vi "FDG Def_Start_Results.vi"(0 "System no.":i32=1 min=1 step=1, 1 "Board":i32=1 min=1 max=5 step=1, 2 "Routinename":string, 5 "error in":errorcluster, 6 "Treshold level":dbl=1.0 format="%.3f", 7 "Frequency settings":cluster{"Set frequency?":bool, "Frequency":dbl}={"Set frequency?"=FALSE, "Frequency"=10.0} {"Frequency" format="%.3f"}, 8 "Velocity settings":cluster{"Set velocity?":bool, "Velocity":dbl}={"Set velocity?"=FALSE, "Velocity"=0.1} {"Velocity" format="%.4f"}, 9 "Max. direction changes settings":T3={"Set max. dir. changes?"=FALSE, "Max. dir. changes"=10}, 10 "Speed factor settings":T4={"Set speed factor?"=FALSE, "Speed factor"=0.25} {"Speed factor" format="%.4f"}, 11 "Speed offset settings":T2={"Set speed offset?"=FALSE, "Speed offset"=0.05} {"Speed offset" format="%.4f"}, 12 "Stop refnum":refnum<vi>, 13 "Polling time in ms":u32=1) -> (14 "Scan successful?":bool, 15 "Level at max. pos.":dbl=1.0 format="%.4f", 16 "Pos. at max. information":string, 19 "error out":errorcluster)   [LabVIEW 2026]
doc: "Defines a fast alignment gradient search routine, starts search, waits until search has finished and queries results. If Stop refnum or Local stop is TRUE, VI sends #24 and stops."
panel:
  in  "Amplitude settings":T1={"Min amplitude"=0.4, "Set min. amplitude?"=FALSE, "Max amplitude"=0.8, "Set max. amplitude?"=FALSE} {"Max amplitude" format="%.4f"; "Min amplitude" format="%.4f"}
  in  "Axis settings":cluster{"Scan axis":string, "Step axis":string}
  in  "Local stop":bool
  # "Defines fast gradient scan, starts scan, waits until scan has finished and queries results.  If Stop refnum or Local stop is TRUE, VI sends #24 and stops."
  # "If Yes:"
  # "If Yes:"
  # "If Yes:"
  # "If Yes:"
  # "If Yes:"
  # "If Yes:"
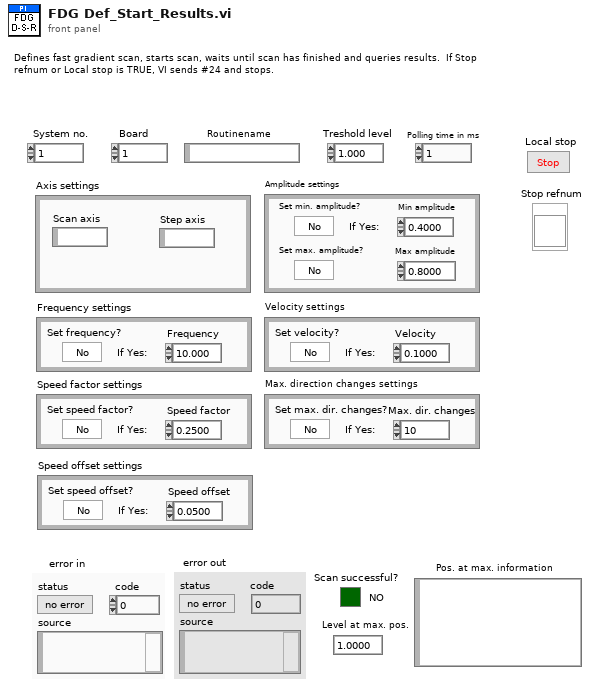
[diagram p1: front panel]
types:
  T1 = cluster{"Min amplitude":dbl, "Set min. amplitude?":bool, "Max amplitude":dbl, "Set max. amplitude?":bool}
  T2 = cluster{"Set speed offset?":bool, "Speed offset":dbl}
  T3 = cluster{"Set max. dir. changes?":bool, "Max. dir. changes":i32}
  T4 = cluster{"Set speed factor?":bool, "Speed factor":dbl}
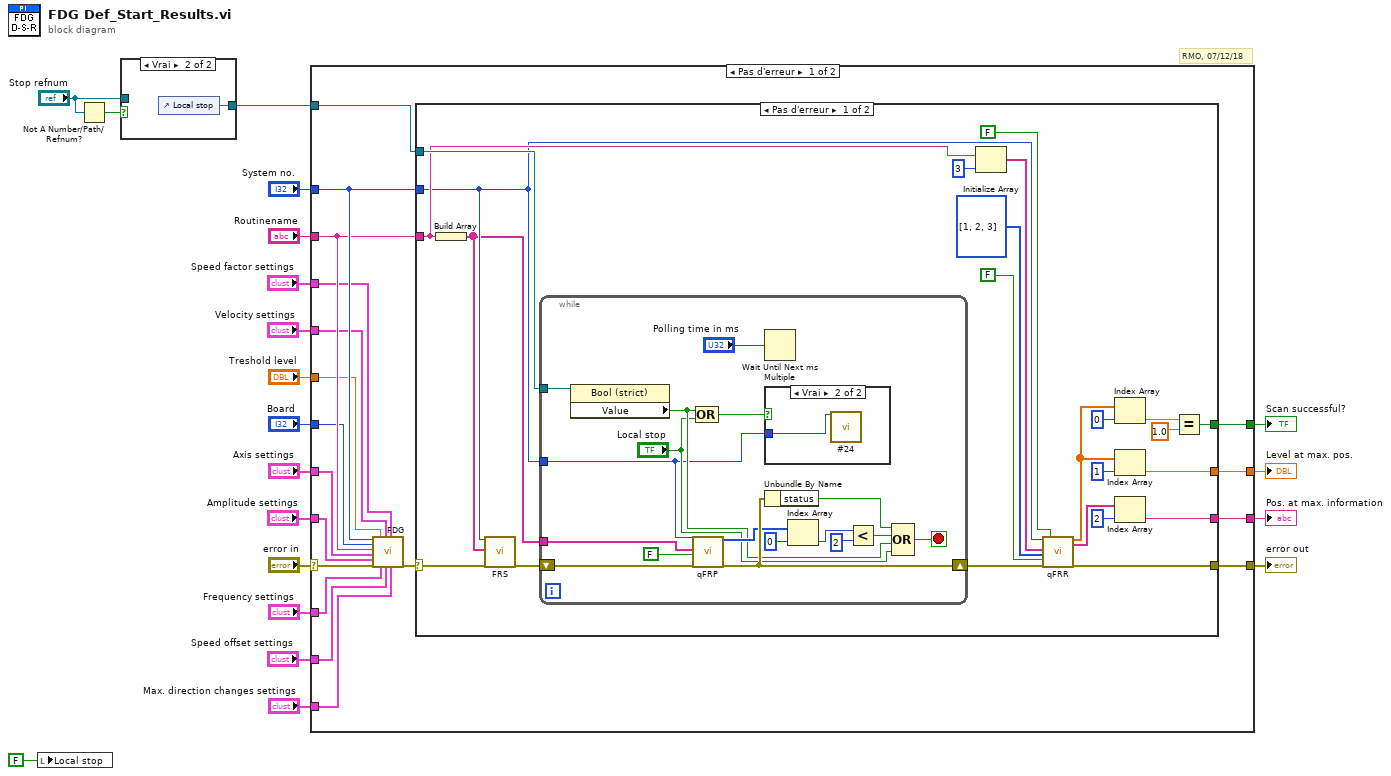
[diagram p0: block diagram]
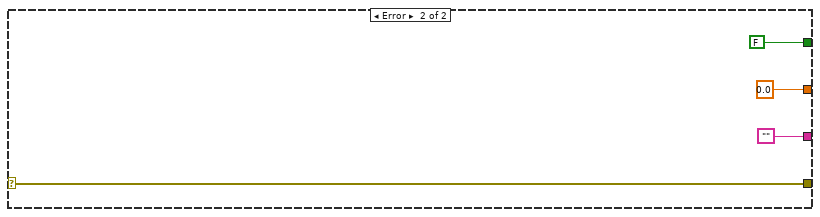
[diagram p4: hidden frame]
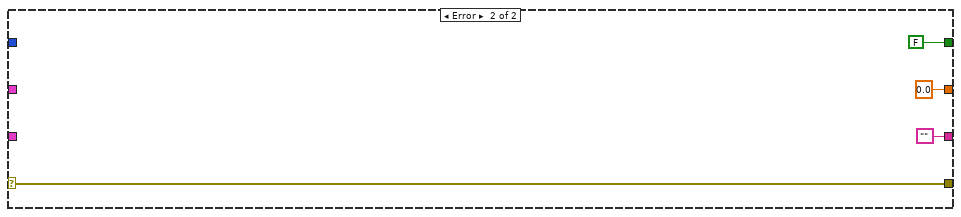
[diagram p5: hidden frame]
diagram:
  # "RMO, 07/12/18"
  n1 = local write "Local stop"(FALSE ("Local stop")) -> ()
  n2 = Not A Number/Path/Refnum?(number/path/refnum="Stop refnum") -> (NaN/Path/Refnum?=w16:bool)
  n3 = case shown="Vrai" w16 {
    tunnel: [w21 w22] -> w15
    tunnel: "Stop refnum" -> [w21 _]
    frame False {
    }
    frame True {
      n4 = control-ref of="Local stop"() -> (w22:refnum<vi>)
    }
  }
  n5 = case shown="Pas d'erreur" "error in" {
    selector: "error in" -> [w23 w86]
    tunnel: [w33 w86] -> w20
    tunnel: [w36 FALSE] -> w19
    tunnel: w15 -> [w39 _]
    tunnel: "System no." -> [w38 _]
    tunnel: "Routinename" -> [w37 _]
    tunnel: [w35 0.0 ("Numeric")] -> w12
    tunnel: [w34 "" ("String")] -> w11
    tunnel: "Board" -> [w32 _]
    tunnel: "Axis settings" -> [w25 _]
    tunnel: "Amplitude settings" -> [w24 _]
    tunnel: "Frequency settings" -> [w31 _]
    tunnel: "Treshold level" -> [w30 _]
    tunnel: "Velocity settings" -> [w29 _]
    tunnel: "Max. direction changes settings" -> [w28 _]
    tunnel: "Speed factor settings" -> [w27 _]
    tunnel: "Speed offset settings" -> [w26 _]
    frame No Error {
      n6 = call "FDG.vi"("System no."=w38, "Board"=w32, "Routinename"=w37, "Axis settings"=w25, "Amplitude settings"=w24, "error in"=w23, "Minimum Level"=w30, "Frequency settings"=w31, "Velocity settings"=w29, "Speed offset settings"=w26, "Speed factor settings"=w27, "Max. direction changes settings"=w28) -> ("error out"=w40:errorcluster)  [unwired: 7 out]
      n7 = case shown="Pas d'erreur" w40 {
        selector: w40 -> [w44 w82]
        tunnel: w39 -> [w63 _]
        tunnel: w38 -> [w42 _]
        tunnel: w37 -> [w59 _]
        tunnel: [w52 FALSE] -> w36
        tunnel: [w50 0.0 ("Numeric")] -> w35
        tunnel: [w46 "" ("String")] -> w34
        tunnel: [w45 w82] -> w33
        frame No Error {
          n8 = Build Array(w59) -> (w41:string[])
          n9 = call "FRS.vi"("System no."=w42, "Routines to start"=w41, "error in"=w44) -> ("error out"=w43:errorcluster)  [unwired: 16 out]
          n10 = while {
            tunnel: w63 -> [w79]
            shift-right: [w76] -> w62
            shift-left: w43 -> [w78]
            tunnel: w42 -> [w65]
            tunnel: w41 -> [w69]
            stop <- w80 stop-if-true
            n11 = property class="Bool (strict)"(reference=w79) -> ("Value"=w68:bool)  [unwired: 1 in, 2 out]
            n12 = call "qFRP.vi"("System no."=w65, "Routines to query"=w69, "All routines?"=FALSE, "error in"=w78) -> ("Status"=w74:i32[], "error out"=w76:errorcluster)  [unwired: 14 out]
            n13 = Compound Arithmetic op=OR(w68, "Local stop") -> (w66:bool)
            n14 = Wait Until Next ms Multiple(millisecond multiple="Polling time in ms") -> ()  [unwired: 1 out]
            n15 = case shown="Vrai" w66 {
              tunnel: w65 -> [_ w81]
              frame False {
              }
              frame True {
                n16 = call "#24.vi"("System no."=w81) -> ()  [unwired: 1 in, 18 out]
              }
            }
            n17 = Unbundle By Name(w76) -> ("status"=w77:bool)
            n18 = Index Array(array=w74, index=0) -> (element=w72:i32)
            n19 = Less?(x=w72, y=2) -> (x < y?=w70:bool)
            n20 = Compound Arithmetic op=OR(w77, w70, w68, "Local stop") -> (w80:bool)
          }
          n21 = Initialize Array(w59, 3 ("dimension size")) -> (w57:string[])
          n22 = call "qFRR.vi"("System no."=w42, "Routinename"=w57, "ResultID"=i32[] [1, 2, 3], "Query all?"=FALSE, "error in"=w62, "Use FRH?"=FALSE) -> ("Value (num.)"=w51:dbl[], "Value (string)"=w47:string[], "error out"=w45:errorcluster)  [unwired: 11 out]
          n23 = Index Array(array=w51, index=0) -> (element=w54:dbl)
          n24 = Index Array(array=w51, index=1) -> (element=w50:dbl)
          n25 = Index Array(array=w47, index=2) -> (element=w46:string)
          n26 = Equal?(x=w54, y=1.0) -> (x = y?=w52:bool)
        }
        frame Error {
        }
      }
    }
    frame Error {
    }
  }
  "error out" <- w20
  "Scan successful?" <- w19
  "Level at max. pos." <- w12
  "Pos. at max. information" <- w11
